vi "Y2subvi.vi"(1 "MAXIMUM":ext format="%.9f", 2 "Variable name":string, 3 "error in (no error)":errorcluster, 4 "MINIMUM":ext format="%.9f", 5 "LIN or LOG axis":string, 6 "VISA resource name":refnum<visa-resource-name>) -> (0 "error out":errorcluster)   [LabVIEW 2012]
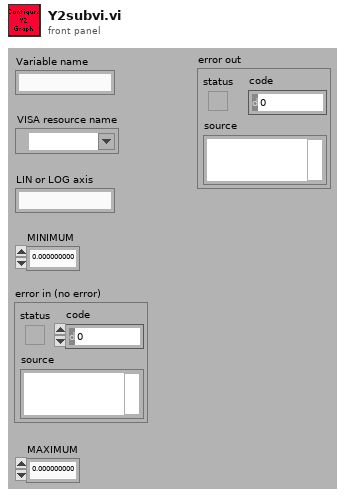
[diagram p1: front panel]
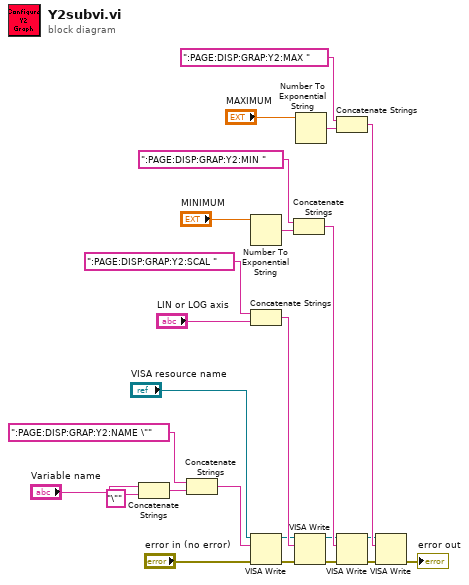
[diagram p0: block diagram]
diagram:
  n1 = Concatenate Strings("Variable name", "\"" ("string")) -> (w3:string)
  n2 = Concatenate Strings(":PAGE:DISP:GRAP:Y2:NAME \"" ("write buffer"), w3) -> (w6:string)
  n3 = Number To Exponential String(number="MINIMUM") -> (E-format string=w18:string)  [unwired: 3 in]
  n4 = Concatenate Strings(":PAGE:DISP:GRAP:Y2:SCAL " ("write buffer"), "LIN or LOG axis") -> (w15:string)
  n5 = VISA Write(VISA resource name="VISA resource name", write buffer=w6, error in (no error)="error in (no error)") -> (VISA resource name out=w7:refnum<visa-resource-name>, error out=w10:errorcluster)  [unwired: 1 out]
  n6 = Concatenate Strings(":PAGE:DISP:GRAP:Y2:MIN " ("write buffer"), w18) -> (w19:string)
  n7 = VISA Write(VISA resource name=w7, write buffer=w15, error in (no error)=w10) -> (VISA resource name out=w8:refnum<visa-resource-name>, error out=w11:errorcluster)  [unwired: 1 out]
  n8 = Number To Exponential String(number="MAXIMUM") -> (E-format string=w20:string)  [unwired: 3 in]
  n9 = Concatenate Strings(":PAGE:DISP:GRAP:Y2:MAX " ("write buffer"), w20) -> (w23:string)
  n10 = VISA Write(VISA resource name=w8, write buffer=w19, error in (no error)=w11) -> (VISA resource name out=w9:refnum<visa-resource-name>, error out=w12:errorcluster)  [unwired: 1 out]
  n11 = VISA Write(VISA resource name=w9, write buffer=w23, error in (no error)=w12) -> (error out=→"error out":errorcluster)  [unwired: 2 out]
